vi "ADS1115_Config_REG.vi"(7 "I2C Slave Address (0) (ADS1115 Address)":u8, 8 "Error In":errorcluster, 9 "options_i2c_write":T1, 10 "ADS1015 Reg Config":T2, 11 "handle":u32) -> (0 "Error Out":errorcluster, 3 "handle out":u32)   [LabVIEW 2017]
uses:
  libMPSSE.lvlib
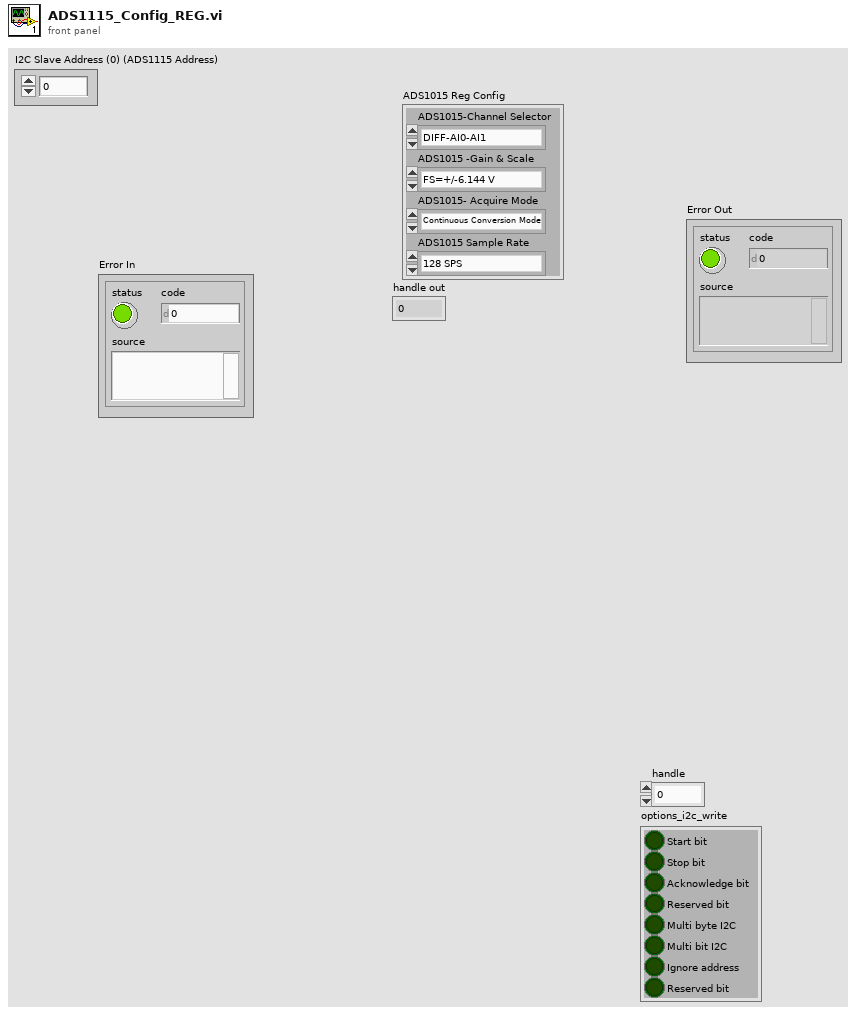
[diagram p1: front panel]
types:
  T1 = cluster{"Start bit":bool, "Stop bit":bool, "Acknowledge bit":bool, "Reserved bit":bool, "Multi byte I2C":bool, "Multi bit I2C":bool, "Ignore address":bool, "Reserved bit":bool}
  T2 = cluster{"ADS1015-Channel Selector":enum8{"DIFF-AI0-AI1", "DIFF-AI0-AI3", "DIFF-AI1-AI3", "DIFF-AI2-AI3", "Single Ended - AI0", "Single Ended - AI1", "Single Ended - AI2", "Single Ended - AI3"}, "ADS1015 -Gain & Scale":enum8{"FS=+/-6.144 V", "FS=+/-4.096 V", "FS=+/-2.048 V", "FS=+/-1.024 V", "FS=+/-0.512 V", "FS=+/-0.256-A V", "FS=+/-0.256-B V", "FS=+/-0.256-C V"}, "ADS1015- Acquire Mode":enum16{"Continuous Conversion Mode", "Single Shot Mode"}, "ADS1015 Sample Rate":enum8{"128 SPS", "250 SPS", "490 SPS", "920 SPS", "1600 SPS", "2400 SPS", "3300 SPS", "3300 SPS A"}}
  T3 = enum8{"DIFF-AI0-AI1", "DIFF-AI0-AI3", "DIFF-AI1-AI3", "DIFF-AI2-AI3", "Single Ended - AI0", "Single Ended - AI1", "Single Ended - AI2", "Single Ended - AI3"}
  T4 = enum8{"FS=+/-6.144 V", "FS=+/-4.096 V", "FS=+/-2.048 V", "FS=+/-1.024 V", "FS=+/-0.512 V", "FS=+/-0.256-A V", "FS=+/-0.256-B V", "FS=+/-0.256-C V"}
  T5 = enum16{"Continuous Conversion Mode", "Single Shot Mode"}
  T6 = enum8{"128 SPS", "250 SPS", "490 SPS", "920 SPS", "1600 SPS", "2400 SPS", "3300 SPS", "3300 SPS A"}
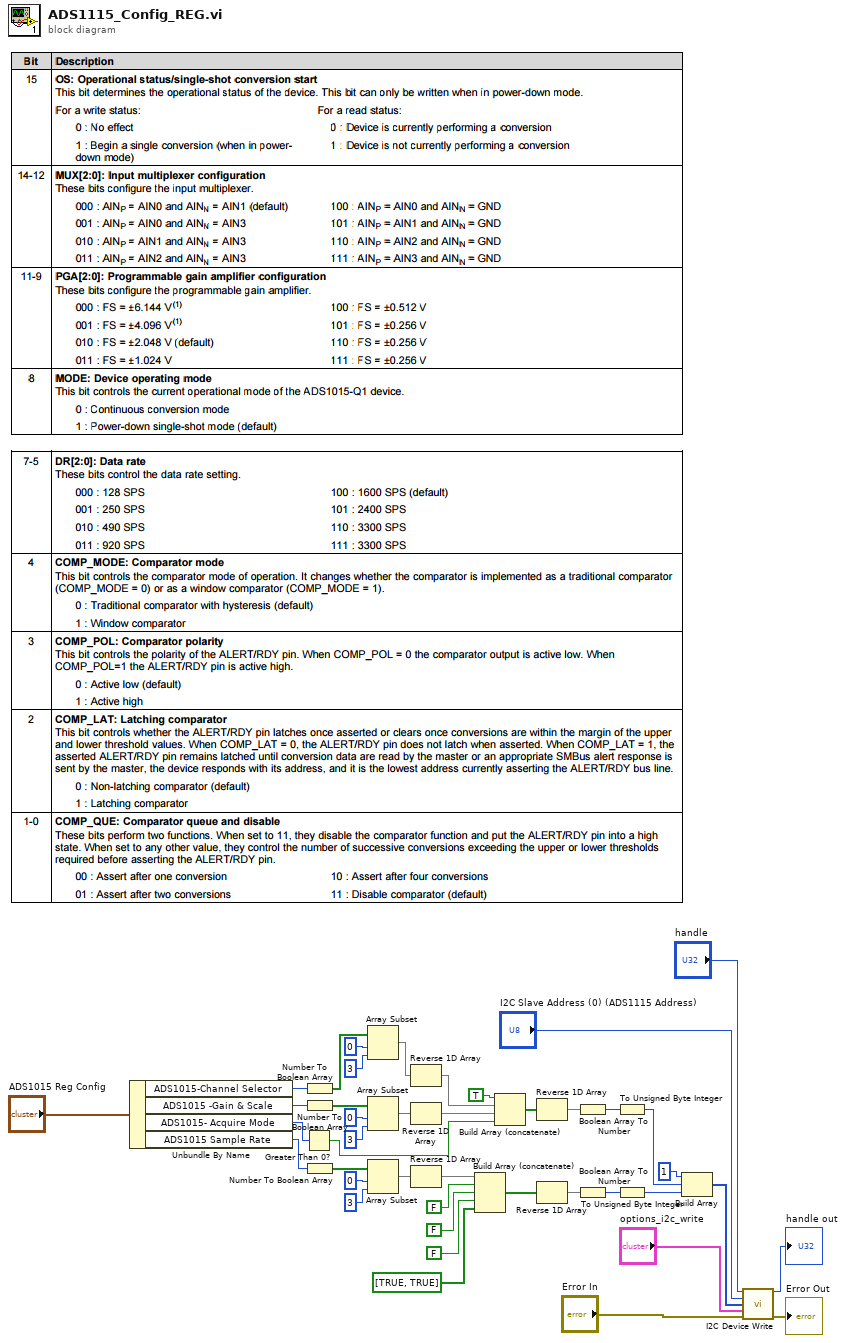
[diagram p0: block diagram]
diagram:
  n1 = Unbundle By Name("ADS1015 Reg Config") -> ("ADS1015-Channel Selector"=w11:T3, "ADS1015 -Gain & Scale"=w10:T4, "ADS1015- Acquire Mode"=w9:T5, "ADS1015 Sample Rate"=w8:T6)
  n2 = Greater Than 0?(x=w9) -> (x > 0?=w16:bool)
  n3 = Number To Boolean Array(number=w11) -> (Boolean array=w27:bool[])
  n4 = Number To Boolean Array(number=w10) -> (Boolean array=w19:bool[])
  n5 = Number To Boolean Array(number=w8) -> (Boolean array=w42:bool[])
  n6 = Array Subset(array=w27, index=0, length=3) -> (w24:bool[])
  n7 = Array Subset(array=w19, index=0, length=3) -> (w18:bool[])
  n8 = Array Subset(array=w42, index=0, length=3) -> (w39:bool[])
  n9 = Reverse 1D Array(array=w24) -> (reversed array=w22:bool[])
  n10 = Reverse 1D Array(array=w18) -> (reversed array=w17:bool[])
  n11 = Reverse 1D Array(array=w39) -> (reversed array=w38:bool[])
  n12 = Build Array (concatenate)(w38, FALSE, FALSE, FALSE, bool[] [TRUE, TRUE] ("array")) -> (w33:bool[])
  n13 = Build Array (concatenate)(TRUE, w22, w17, w16) -> (w15:bool[])
  n14 = Reverse 1D Array(array=w15) -> (reversed array=w14:bool[])
  n15 = Reverse 1D Array(array=w33) -> (reversed array=w32:bool[])
  n16 = Boolean Array To Number(Boolean array=w14) -> (number=w13:u32)
  n17 = Boolean Array To Number(Boolean array=w32) -> (number=w31:u32)
  n18 = To Unsigned Byte Integer(number=w13) -> (unsigned 8bit integer=w30:u8)
  n19 = To Unsigned Byte Integer(number=w31) -> (unsigned 8bit integer=w28:u8)
  n20 = Build Array(u8 1 ("element"), w30, w28) -> (w7:u8[])
  n21 = call "I2C Device Write.vi"("handle"="handle", "deviceAddress"="I2C Slave Address (0) (ADS1115 Address)", "Data to write"=w7, "options"="options_i2c_write", "error in (no error)"="Error In") -> ("handle out"=→"handle out":u32, "error out"=→"Error Out":errorcluster)  [unwired: 8 in, 1 out]
